vi "Coerce to Enum__ogtk.vi"   [LabVIEW 2012]
doc: "This is a merged VI which will place appropriate code for coersion from numeric to an enum"
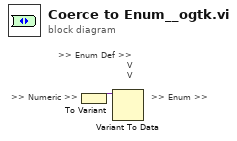
[diagram p0: block diagram]
diagram:
  # ">> Enum >>"
  # ">> Enum Def >>\n                       V\n                       V"
  # ">> Numeric >>"
  n1 = To Variant() -> (Variant=w1:variant)  [unwired: 1 in]
  n2 = Variant To Data(Variant=w1) -> ()  [unwired: 2 in, 2 out]
